vi "FrontPanelMenu.vi"() -> ()   [LabVIEW 2018]
panel:
  in  "?":bool
  out "Waveform Chart":dbl[](graph)
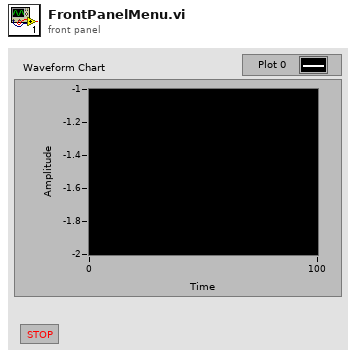
[diagram p1: front panel]
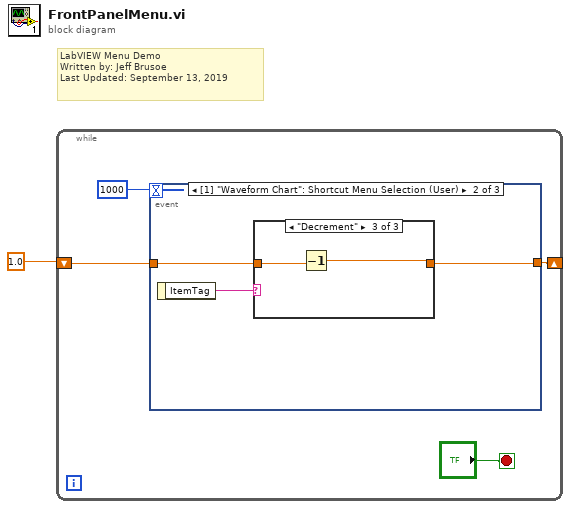
[diagram p0: block diagram]
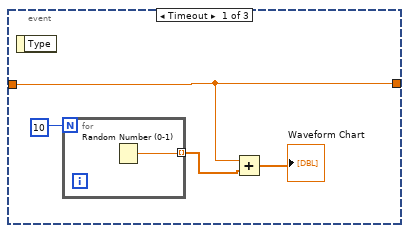
[diagram p2: hidden frame]
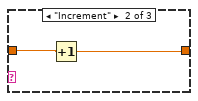
[diagram p4: hidden frame]
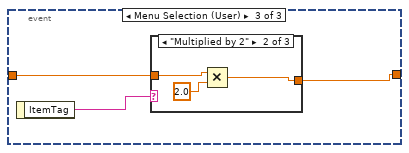
[diagram p5: hidden frame]
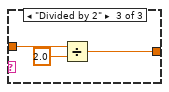
[diagram p7: hidden frame]
diagram:
  # "LabVIEW Menu Demo\nWritten by: Jeff Brusoe\nLast Updated: September 13, 2019"
  n1 = while {
    shift-right: [w2] -> _
    shift-left: 1.0 -> [w3]
    stop <- "?" stop-if-true
    n2 = event shown="[1] \"Waveform Chart\": Shortcut Menu Selection (User)" {
      selector: _ -> [_ _ _]
      dyn-events: _ -> [_ _ _]
      timeout: 1000 -> [_ _ _]
      tunnel: w3 -> [w8 w12 w20]
      tunnel: [w8 w11 w19] -> w2
      event Timeout {
        n3 = event-data() -> ()  [unwired: 1 in, 1 out]
        n4 = for {
          N: 10 -> [_]
          tunnel: [w10] -> w6 mode=indexing
          n5 = Random Number (0-1)() -> (number: 0 to 1=w10:dbl)
        }
        n6 = Add(x=w8, y=w6) -> (x+y=→"Waveform Chart":dbl[])
      }
      event "Waveform Chart": Shortcut Menu Selection (User) {
        n7 = event-data() -> ("ItemTag"=w13:string)  [unwired: 1 in]
        n8 = case shown="\"Decrement\"" w13 {
          tunnel: w12 -> [w14 w16 w18]
          tunnel: [w14 w15 w17] -> w11
          frame Default {
          }
          frame "Increment" {
            n9 = Increment(x=w16) -> (x+1=w15:dbl)
          }
          frame "Decrement" {
            n10 = Decrement(x=w18) -> (x-1=w17:dbl)
          }
        }
      }
      event Menu Selection (User) {
        n11 = event-data() -> ("ItemTag"=w21:string)  [unwired: 1 in]
        n12 = case shown="\"Multiplied by 2\"" w21 {
          tunnel: w20 -> [w22 w25 w28]
          tunnel: [w22 w23 w26] -> w19
          frame Default {
          }
          frame "Multiplied by 2" {
            n13 = Multiply(x=w25, y=2.0) -> (x*y=w23:dbl)
          }
          frame "Divided by 2" {
            n14 = Divide(x=w28, y=2.0) -> (x/y=w26:dbl)
          }
        }
      }
    }
  }
